vi "Data_Acquisition.vi"(5 "start Datetime":cluster{"row":i32, "column":i32}={"row"=1, "column"=0}, 7 "end Datetime":cluster{"row":i32, "column":i32}={"row"=3504, "column"=0}, 9 "start Data":cluster{"start row":i32, "start column":i32}={"start row"=1, "start column"=1}, 11 "end Data":cluster{"row":i32, "column":i32}={"row"=3504, "column"=4}) -> (8 "Meas":T1)   [LabVIEW 2022 SP3]
uses:
  <vilib>/Utility/NIReport.llb/Report Type.ctl
  <vilib>/addons/_office/excel.llb/Excel Get Data ([str]).vi
  <vilib>/addons/_office/excel.llb/Excel Get Data ([dbl]).vi
  <vilib>/Utility/NIReport.llb/NI_report.lvclass
  <vilib>/addons/_office/NI_ReportGenerationToolkit.lvlib
  <vilib>/Utility/NIReport.llb/NI_ReportGenerationCore.lvlib
  <vilib>/Utility/NIReport.llb/Excel/NI_Excel.lvclass
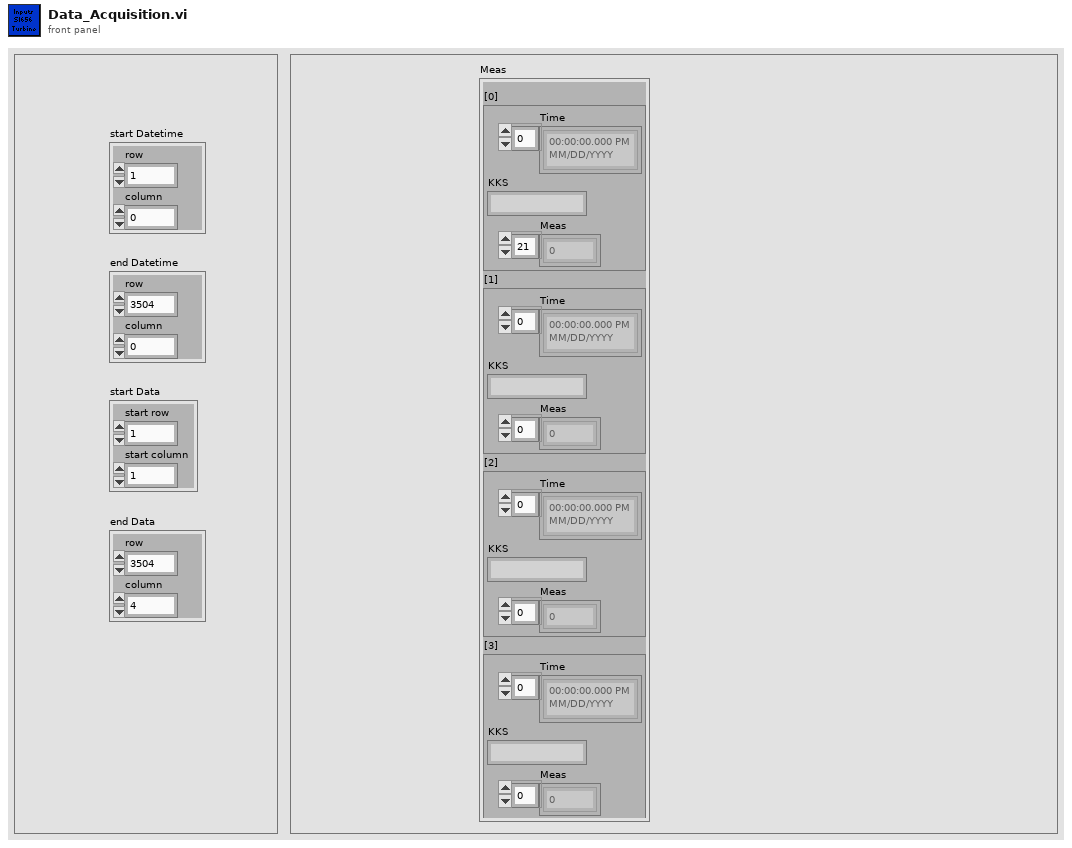
[diagram p1: front panel]
types:
  T1 = cluster{"[0]":cluster{"Time":timestamp[], "KKS":string, "Meas":dbl[]}, "[1]":cluster{"Time":timestamp[], "KKS":string, "Meas":dbl[]}, "[2]":cluster{"Time":timestamp[], "KKS":string, "Meas":dbl[]}, "[3]":cluster{"Time":timestamp[], "KKS":string, "Meas":dbl[]}, "[4]":cluster{"Time":timestamp[], "KKS":string, "Meas":dbl[]}, "[5]":cluster{"Time":timestamp[], "KKS":string, "Meas":dbl[]}, "[6]":cluster{"Time":timestamp[], "KKS":string, "Meas":dbl[]}, "[7]":cluster{"Time":timestamp[], "KKS":string, "Meas":dbl[]}, "[8]":cluster{"Time":timestamp[], "KKS":string, "Meas":dbl[]}}
  T2 = enum16{"maximized", "minimized", "normal", "no change"}
  T3 = cluster{"Time":timestamp[], "KKS":string, "Meas":dbl[]}
  T4 = cluster{"Time":timestamp[], "KKS":string, "Meas":dbl[]}[]
  T5 = typedef "NI_ReportGenerationCore.lvlib/Report Type.ctl" = enum16{"HTML", "Word", "Excel"}
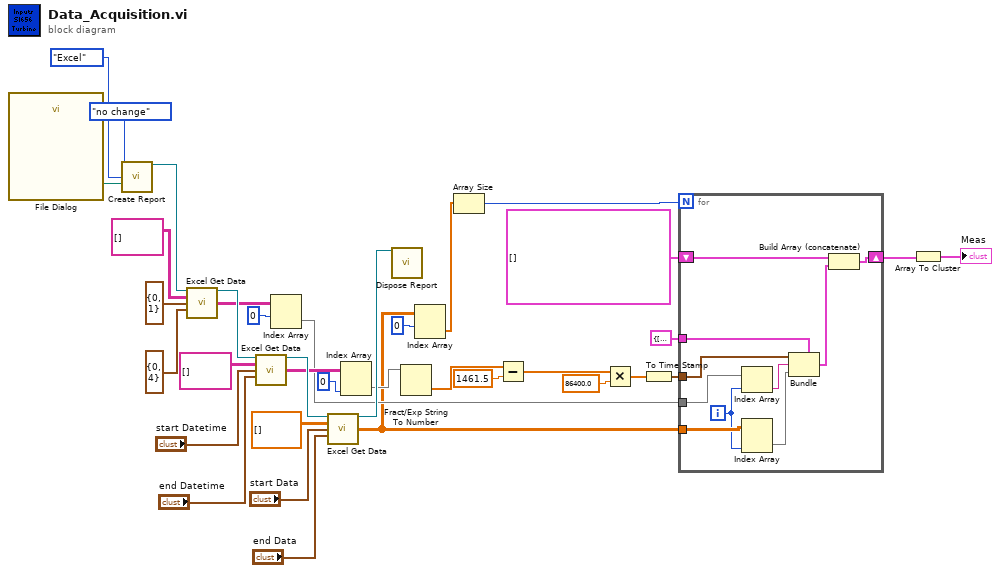
[diagram p0: block diagram]
diagram:
  n1 = call "File Dialog"() -> ("selected path"=w31:path)  [unwired: 12 in, 3 out]
  n2 = call <vilib>:"Create Report.vi"("window state (normal)"=T2."no change", "report type"=Report_Type."Excel", "template (empty)"=w31) -> ("report out"=w18:refnum<class "NI_report.lvclass">)  [unwired: 11 in, 1 out]
  n3 = call-poly <vilib>:"Excel Get Data.vi"("report in"=w18, "data type"=string[][] [], "start (-1, -1)"=cluster{"start row":i32, "start column":i32} {"start row"=0, "start column"=1} ("start (0, 0)"), "end (-1, -1)"=cluster{"row":i32, "column":i32} {"row"=0, "column"=4}) -> ("report out"=w17:refnum<class "NI_report.lvclass">, "data"=w11:string[][])  [unwired: 9 in, 1 out]
  n4 = call-poly <vilib>:"Excel Get Data.vi"("report in"=w17, "data type"=string[][] [], "start (-1, -1)"="start Datetime", "end (-1, -1)"="end Datetime") -> ("report out"=w27:refnum<class "NI_report.lvclass">, "data"=w21:string[][])  [unwired: 9 in, 1 out]
  n5 = Index Array(array=w11, index (row)=0) -> (element=w9:string[])  [unwired: 1 in]
  n6 = call-poly <vilib>:"Excel Get Data.vi"("report in"=w27, "data type"=dbl[][] [], "start (-1, -1)"="start Data", "end (-1, -1)"="end Data") -> ("report out"=w33:refnum<class "NI_report.lvclass">, "data"=w7:dbl[][])  [unwired: 9 in, 1 out]
  n7 = Index Array(array=w21, index (col)=0 ("disabled index (col)")) -> (element=w19:string[])  [unwired: 1 in]
  n8 = call-dynamic "Dispose Report.vi"("report in"=w33) -> ()  [unwired: 14 in, 1 out]
  n9 = Fract/Exp String To Number(string=w19) -> (number=w26:dbl[])  [unwired: 3 in, 1 out]
  n10 = Index Array(array=w7, index (row)=0) -> (element=w5:dbl[])  [unwired: 1 in]
  n11 = Array Size(array=w5) -> (size(s)=w4:i32)
  n12 = Subtract(x=w26, y=1461.5) -> (x-y=w24:dbl[])
  n13 = Multiply(x=w24, y=86400.0) -> (x*y=w22:dbl[])
  n14 = To Time Stamp(1:w22) -> (0:w13:timestamp[])
  n15 = for {
    N: w4 -> [_]
    tunnel: w9 -> [w46]
    tunnel: w7 -> [w39]
    tunnel: w13 -> [w41]
    shift-right: [w43] -> w3
    shift-left: T4 [] -> [w42]
    tunnel: T3 {"Time"=[], "KKS"="", "Meas"=[]} -> [w40]
    i -> [w37]
    n16 = Index Array(array=w46, index=w37) -> (element=w45:string)
    n17 = Index Array(array=w39, index (col)=w37) -> (element=w38:dbl[])  [unwired: 1 in]
    n18 = Bundle(cluster=w40, "Time"=w41, "KKS"=w45, "Meas"=w38) -> (w44:T3)
    n19 = Build Array (concatenate)(w42, w44) -> (w43:T4)
  }
  n20 = Array To Cluster(array=w3) -> (cluster=→"Meas":T1)
